vi "Image_Creator.vi"(6 "Image Data Type":u8=44 format="%x", 7 "Pattern":enum16{"24 Color Checker", "Customized Pure"}(ring)=enum."Customized Pure", 8 "error in (no error)":errorcluster, 9 "Bayer Pattern":T3, 10 "Image Configuration":T4={"Width"=1920, "Height"=1080}, 11 "Pure Color Pattern Parameters":cluster{"R":u8, "G":u8, "B":u8}={"R"=255, "G"=255, "B"=255}) -> (0 "error out":errorcluster, 1 "Image Data Config":T1={"Lines of Image Data"=0, "Bytes per Even Line"=0, "Bytes per Odd Line"=0, "Image Data Type"=44, "Total Image Data Block Size"=0, "Image Data Block Offset"=0} {"Image Data Type" format="%x"}, 2 "Image":T2(plugin-control), 3 "Image Data Payload (U8)":u8[](array[numeric]))   [LabVIEW 2020]
uses:
  ctl/Image_Configuration.ctl
  ctl/Image_RAW_Bayer_Pattern.ctl
  ctl/Image_Data_Config.ctl
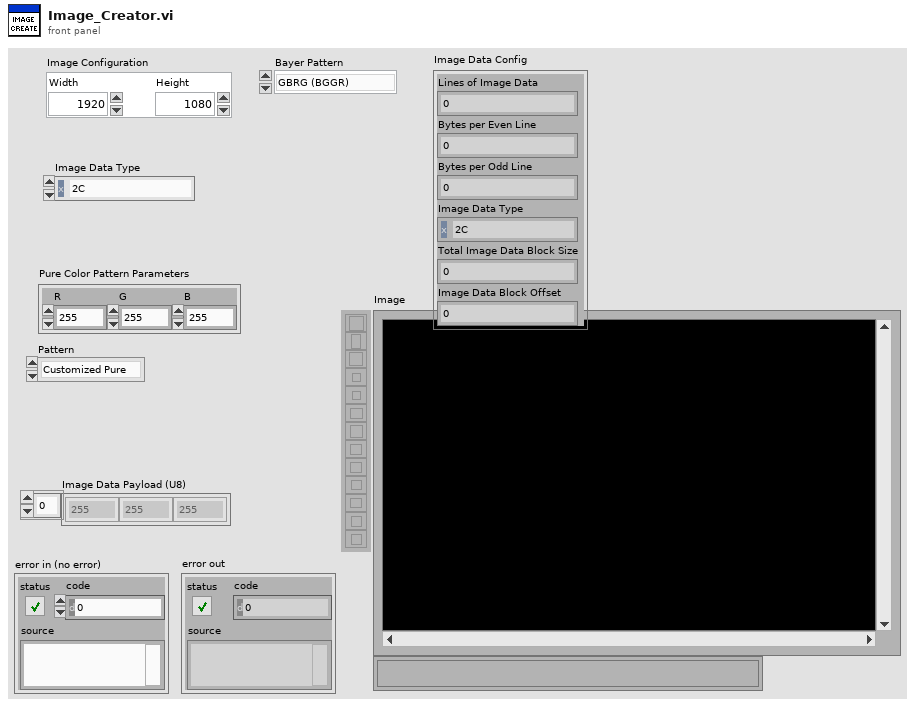
[diagram p1: front panel]
types:
  T1 = typedef "Image_Data_Config.ctl" = cluster{"Lines of Image Data":u16, "Bytes per Even Line":u16, "Bytes per Odd Line":u16, "Image Data Type":u8, "Total Image Data Block Size":u32, "Image Data Block Offset":u32}
  T2 = typedef "IMAQ Image.ctl" = refnum<image>
  T3 = typedef "Image_RAW_Bayer_Pattern.ctl" = enum16{"GBRG (BGGR)", "GRBG (RGGB)", "BGGR (GBRG)", "RGGB (GRBG)", "CRBC (RCCB)"}
  T4 = typedef "Image_Configuration.ctl" = cluster{"Width":i32, "Height":i32}
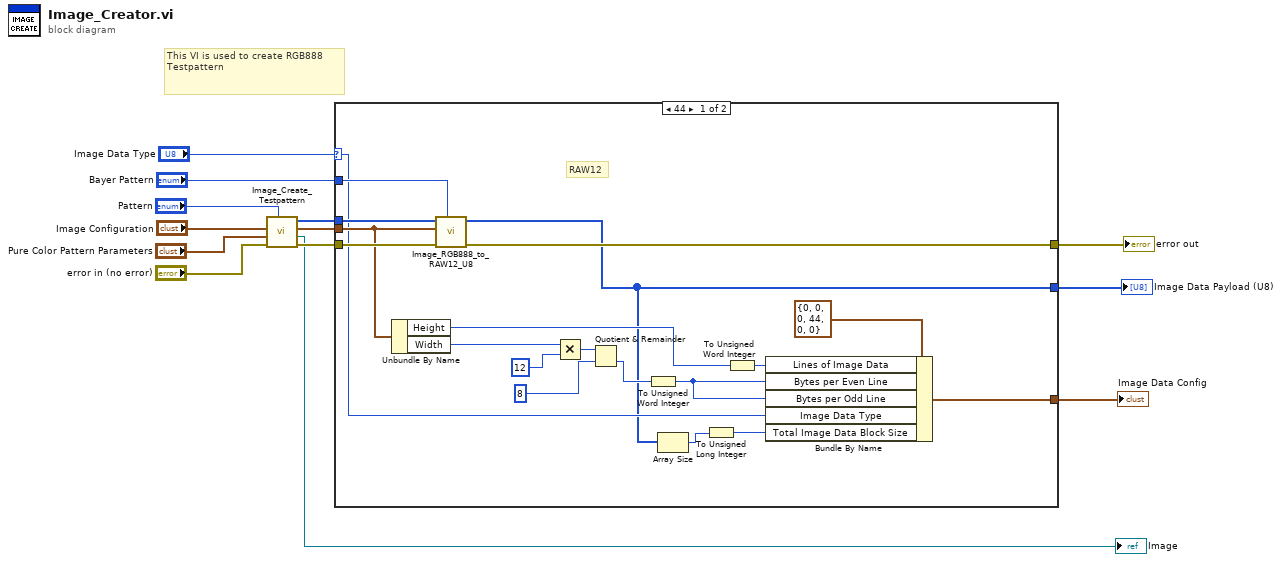
[diagram p0: block diagram]
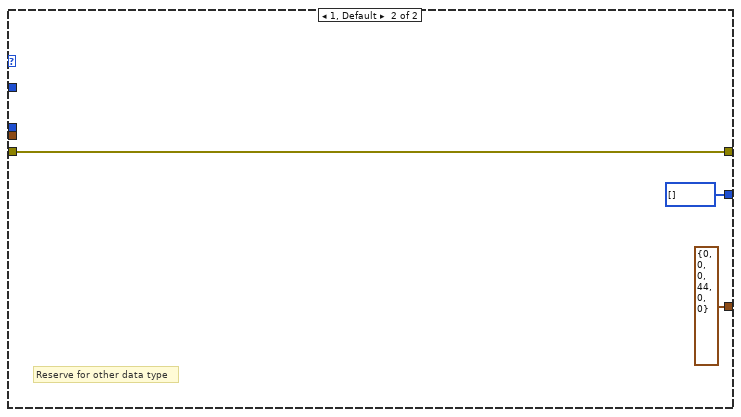
[diagram p2: hidden frame]
diagram:
  # "This VI is used to create RGB888 Testpattern"
  n1 = call "Image_Create_Testpattern.vi"("Pattern"="Pattern", "error in (no error)"="error in (no error)", "Pure Color Pattern Parameters"="Pure Color Pattern Parameters", "Image Configuration"="Image Configuration") -> ("error out"=w10:errorcluster, "Image"=→"Image":T2, "Image Configuration Out"=w7:T4, "RGB U8"=w11:u8[])  [unwired: 4 in]
  n2 = case shown="44" "Image Data Type" {
    selector: "Image Data Type" -> [w18 _]
    tunnel: w11 -> [w32 _]
    tunnel: w10 -> [w31 w33]
    tunnel: [w17 u8[] [] ("RAW12 Frame (U8)")] -> w8
    tunnel: w7 -> [w28 _]
    tunnel: "Bayer Pattern" -> [w30 _]
    tunnel: [w29 w33] -> w5
    tunnel: [w14 T1 {"Lines of Image Data"=0, "Bytes per Even Line"=0, "Bytes per Odd Line"=0, "Image Data Type"=44, "Total Image Data Block Size"=0, "Image Data Block Offset"=0} ("Image Data Config")] -> w2
    frame 44 {
      # "RAW12"
      n3 = Unbundle By Name(w28) -> ("Height"=w21:i32, "Width"=w27:i32)
      n4 = call "Image_RGB888_to_RAW12_U8.vi"("Bayer Pattern"=w30, "error in (no error)"=w31, "Image Configuration"=w28, "RGB Frame (U8)"=w32) -> ("error out"=w29:errorcluster, "RAW12 Frame (U8)"=w17:u8[])  [unwired: 6 in]
      n5 = Multiply(x=w27, y=12) -> (x*y=w25:i32)
      n6 = Quotient & Remainder(x=w25, y=8) -> (floor(x/y)=w20:i32)  [unwired: 1 out]
      n7 = To Unsigned Word Integer(number=w20) -> (unsigned 16bit integer=w19:u16)
      n8 = Array Size(array=w17) -> (size(s)=w16:i32)
      n9 = To Unsigned Long Integer(number=w16) -> (unsigned 32bit integer=w15:u32)
      n10 = To Unsigned Word Integer(number=w21) -> (unsigned 16bit integer=w23:u16)
      n11 = Bundle By Name(cluster=T1 {"Lines of Image Data"=0, "Bytes per Even Line"=0, "Bytes per Odd Line"=0, "Image Data Type"=44, "Total Image Data Block Size"=0, "Image Data Block Offset"=0} ("Image Data Config"), "Lines of Image Data"=w23, "Bytes per Even Line"=w19, "Bytes per Odd Line"=w19, "Image Data Type"=w18, "Total Image Data Block Size"=w15) -> (w14:T1)
    }
    frame 1, Default {
      # "Reserve for other data type"
    }
  }
  "error out" <- w5
  "Image Data Payload (U8)" <- w8
  "Image Data Config" <- w2
